vi "PLC.Dial800.Build OPC Browse and Test Value.vi"() -> ()   [LabVIEW 2018]
panel:
  out "quality":u64
  out "status":u32
  out "Value":bool
  in  "Browse":bool
  out "error out":errorcluster
  out "URL":string="opc://localhost/RSLinx OPC Server/[Stn800]Program:Stn001_90_OffloadMain.TestPC[0].Done"
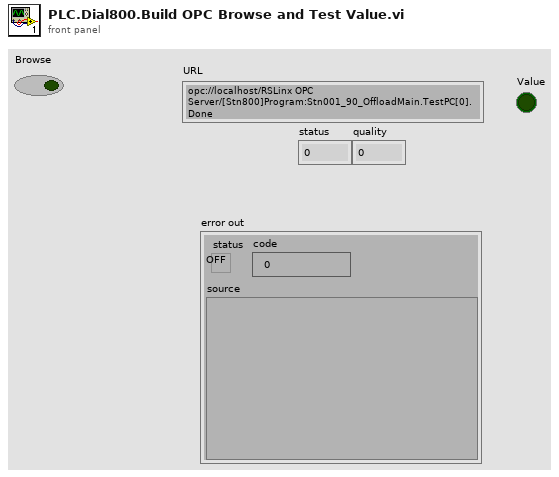
[diagram p1: front panel]
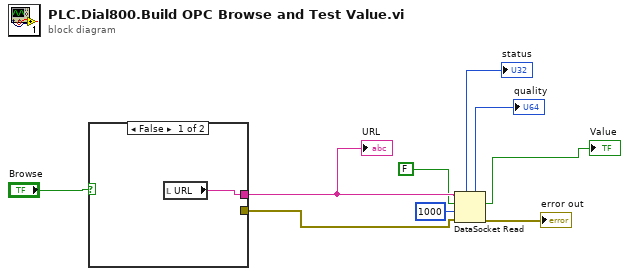
[diagram p0: block diagram]
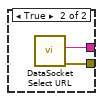
[diagram p2: hidden frame]
diagram:
  n1 = case shown="False" "Browse" {
    tunnel: [w10 w12] -> w9
    tunnel: [_ w11] -> w5
    frame False {
      n2 = local read "URL"() -> (w10:string)
    }
    frame True {
      n3 = call <vilib>:"DataSocket Select URL.vi"() -> ("error out"=w11:errorcluster, "URL"=w12:string)  [unwired: 9 in, 1 out]
    }
  }
  "URL" <- w9
  n4 = DataSocket Read(8:w5, 9:1000 ("ms timeout (10000)"), 10:FALSE, 11:w9) -> (0:→"error out":errorcluster, 2:→"Value":bool, 5:→"quality":u64, 7:→"status":u32)  [unwired: 1 in, 3 out]
